vi "Autonomous Play Globals.vi"() -> ()   [LabVIEW 2015]
panel:
  out "Filepath Array":string[](array[string])
  in  "FileName Array":string[](array[string])
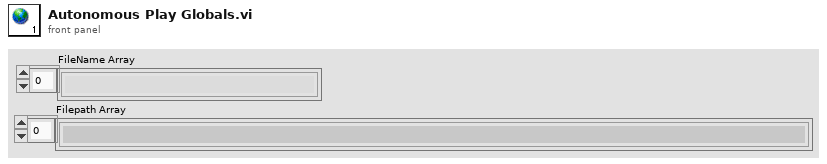
[diagram p1: front panel]
diagram:
